vi "write_params.vi"(8 "error in (no error)":errorcluster, 10 "prams":T1={"eps"=0.5, "min_samples"=5.0, "metric"="euclidean", "algorithm"="auto", "leaf_size"=30.0, "p"=2.0, "n_jobs"=1.0}, 11 "DBSCAN in":refnum<class "DBSCAN.lvclass">) -> (0 "error out":errorcluster, 3 "DBSCAN out":refnum<class "DBSCAN.lvclass">)   [LabVIEW 2020, in "DBSCAN.lvclass"]
uses:
  DBSCAN.lvclass
  Controls/dbscan_params.ctl
  DBSCAN.lvclass/DBSCAN.ctl
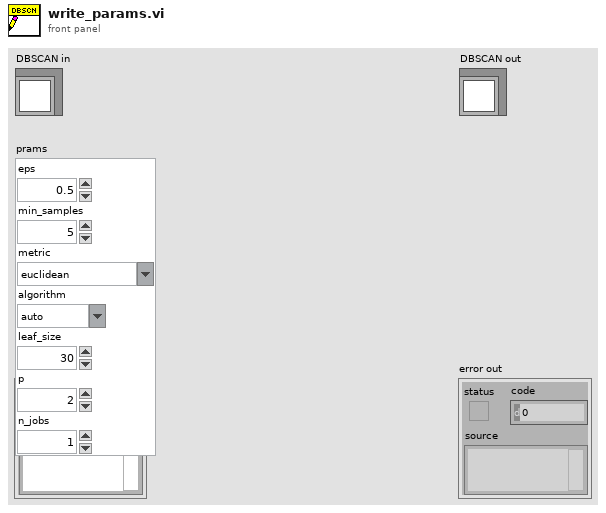
[diagram p1: front panel]
types:
  T1 = typedef "dbscan_params.ctl" = cluster{"eps":dbl, "min_samples":dbl, "metric":string, "algorithm":string, "leaf_size":dbl, "p":dbl, "n_jobs":dbl}
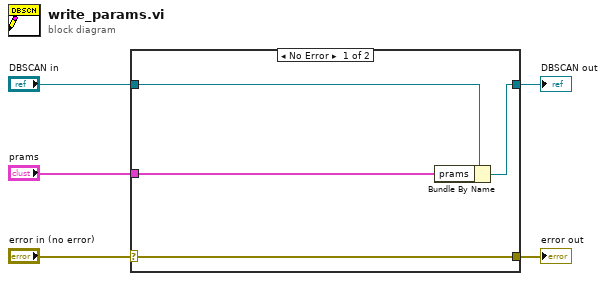
[diagram p0: block diagram]
diagram:
  n1 = case shown="No Error" "error in (no error)" {
    selector: "error in (no error)" -> [w9 w10]
    tunnel: [w9 w10] -> w4
    tunnel: [w7 w11] -> w2
    tunnel: "DBSCAN in" -> [w8 w11]
    tunnel: "prams" -> [w6 _]
    frame No Error {
      n2 = Bundle By Name(cluster=w8, "prams"=w6) -> (w7:refnum<class "DBSCAN.lvclass">)
    }
    frame Error {
    }
  }
  "error out" <- w4
  "DBSCAN out" <- w2
